vi "Lock VIs_V2.vi"() -> ()   [LabVIEW 2024]
panel:
  out "Errors":T1(array[cluster])
  in  "UnProtect All":bool
  in  "Protect All":bool
  out "Busy":bool
  in  "Reset":bool
  in  "Files":T2(array[cluster]) caption="Folder                                                                                Name                             Protected        Protect"
  in  "Unlock":bool
  in  "Lock":bool
  in  "Get Files":bool
  out "Locked Cnt":i32
  in  "Lock PW":string="KwestEng#8002"
  in  "Unlock PW":string
  in  "Folder":path
  # "Lock VIs Utility"
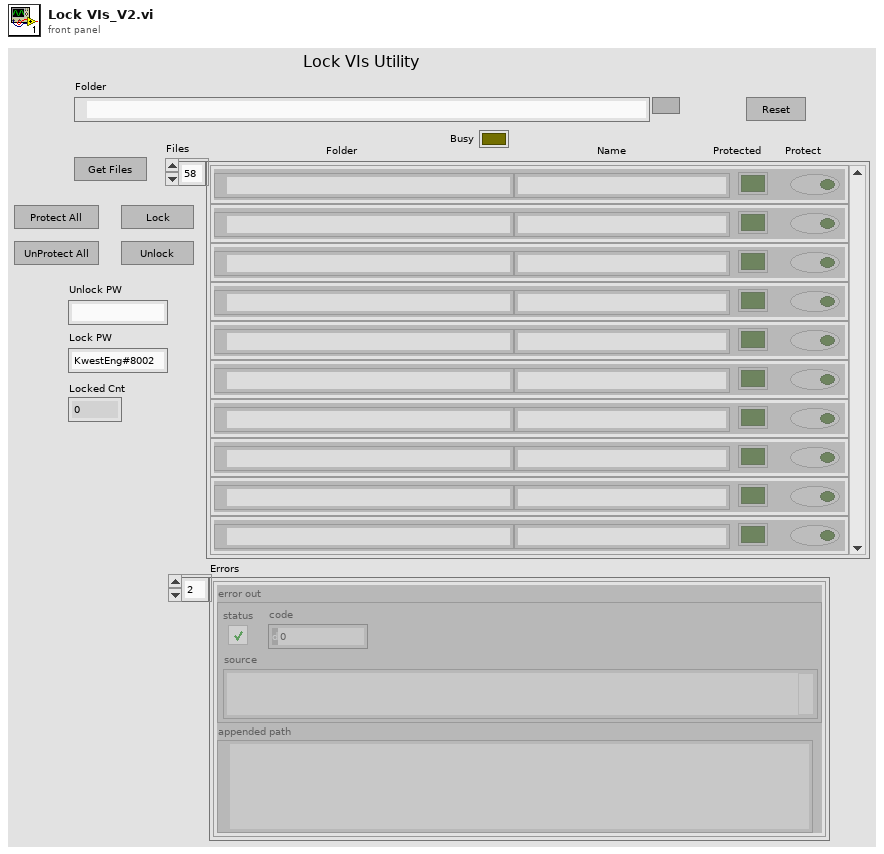
[diagram p1: front panel]
types:
  T1 = cluster{"error out":errorcluster, "appended path":path}[]
  T2 = cluster{"Name":string, "Folder":path, "Status":bool, "Protect":bool}[]
  T3 = enum32{"invalid app kind", "Development System", "Run Time System", "Student Edition", "Embedded LabVIEW", "Evaluation", "Custom"}
  T4 = cluster{"Name":string, "Folder":path, "Status":bool, "Protect":bool}
  T5 = enum32{"invalid lock state", "Not Locked", "Locked (No Password)", "Password-protected"}
  T6 = cluster{"Files":cluster{"Name":string, "Folder":path, "Status":bool, "Protect":bool}[], "UnlockPW":string, "LockPW":string}
  T7 = enum8{"Enabled", "Disabled", "Disabled and Grayed Out"}
  T8 = cluster{"error out":errorcluster, "appended path":path}
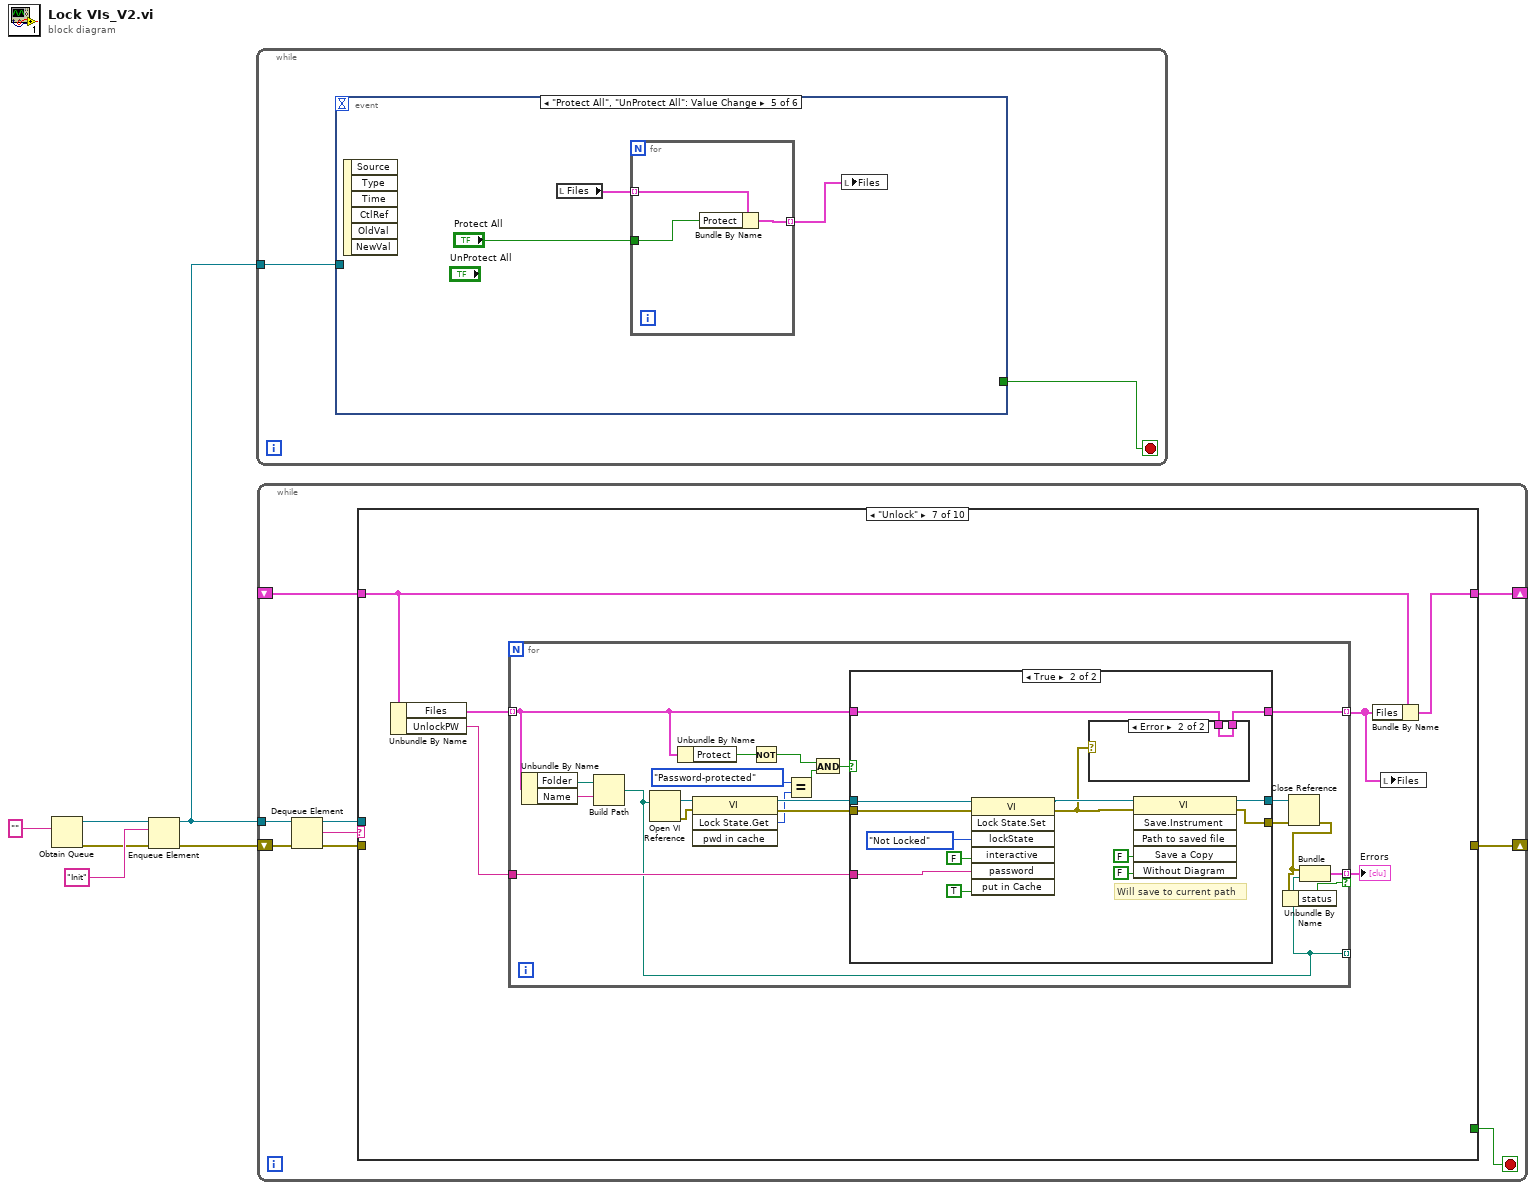
[diagram p0: block diagram]
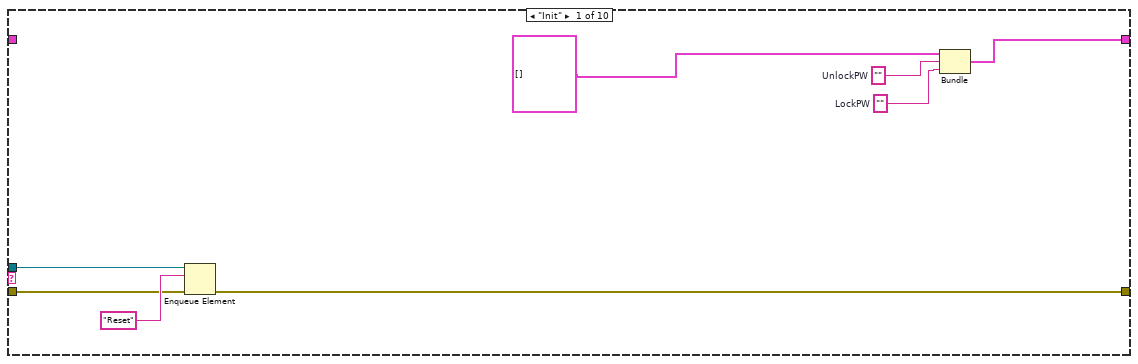
[diagram p2: hidden frame]
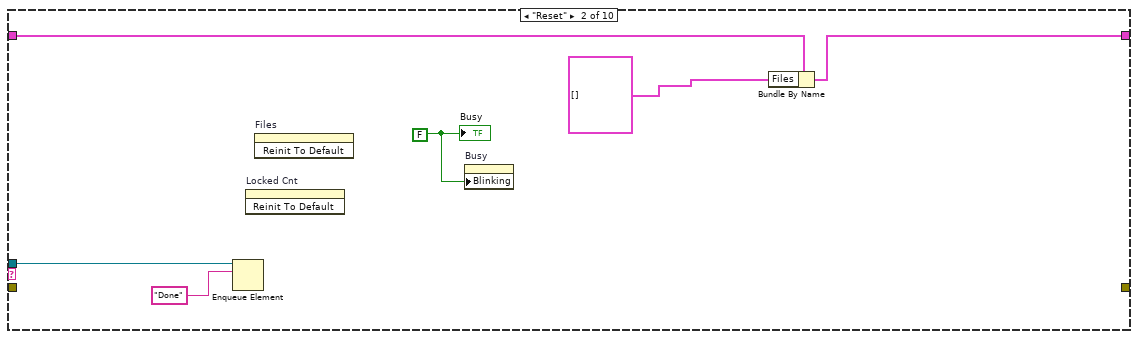
[diagram p3: hidden frame]
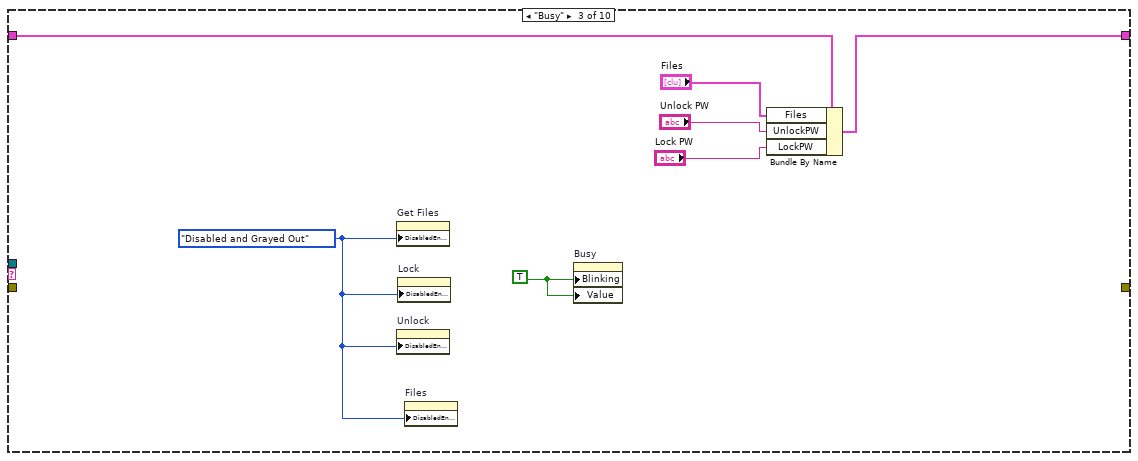
[diagram p4: hidden frame]
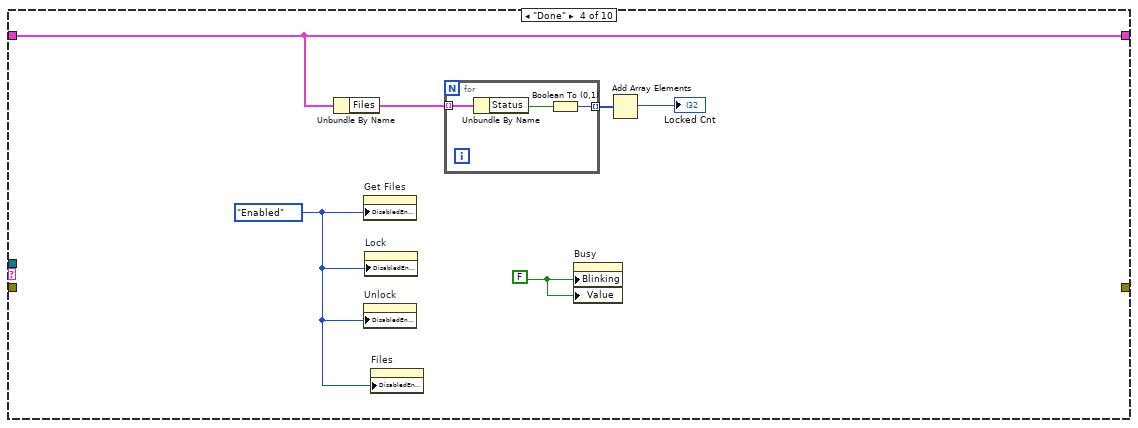
[diagram p5: hidden frame]
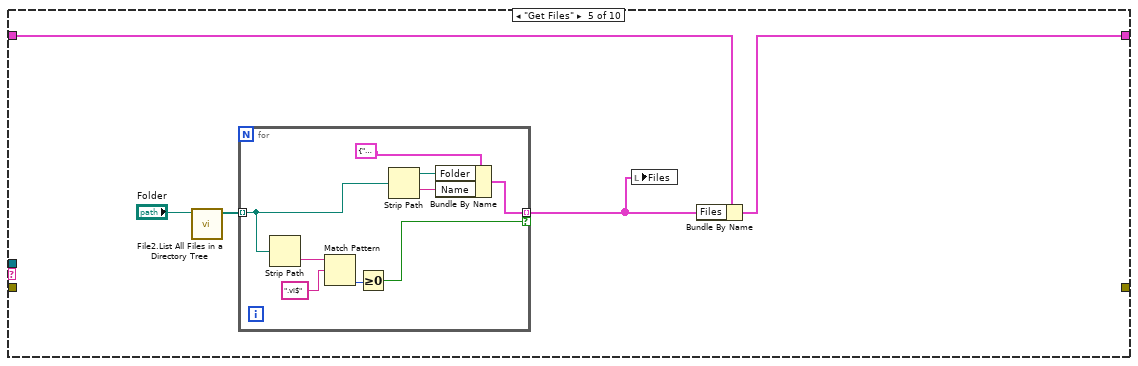
[diagram p6: hidden frame]
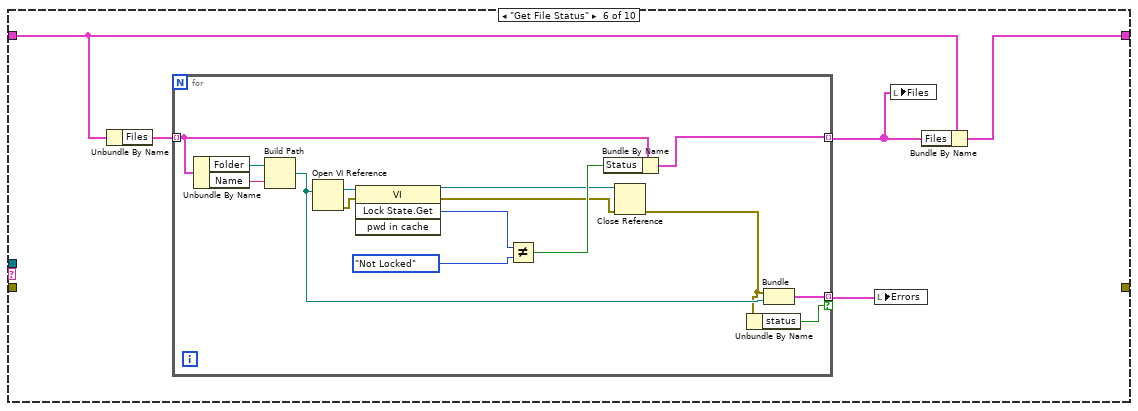
[diagram p7: hidden frame]
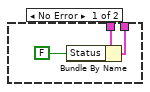
[diagram p9: hidden frame]
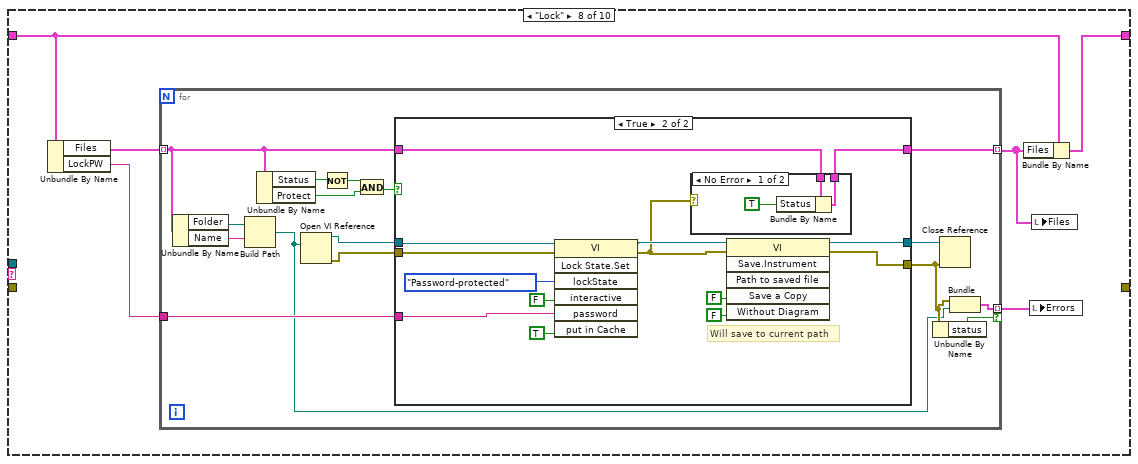
[diagram p10: hidden frame]
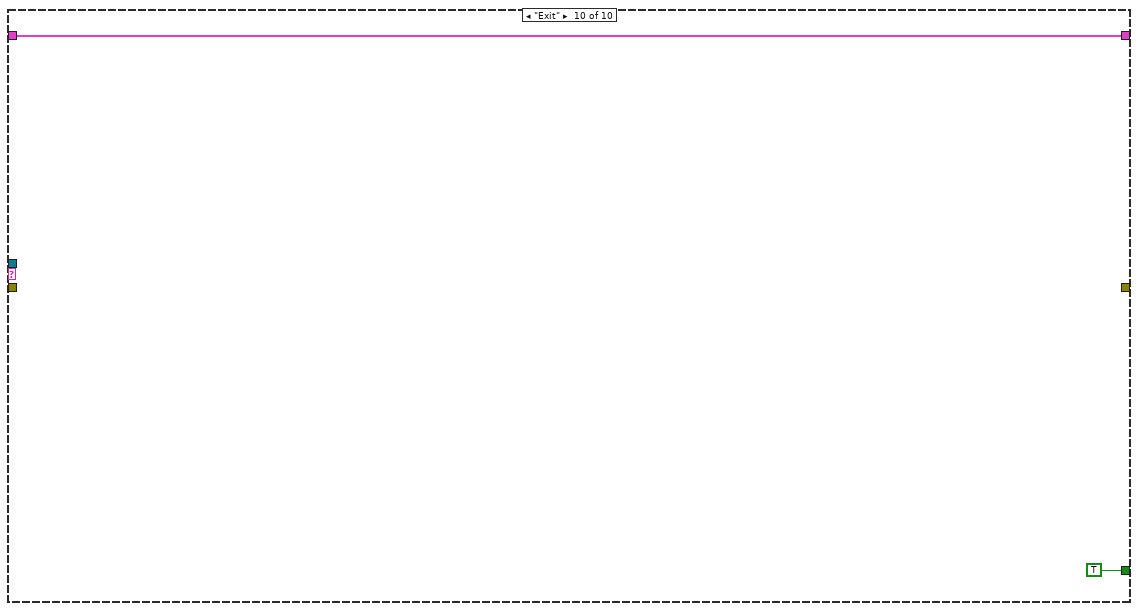
[diagram p14: hidden frame]
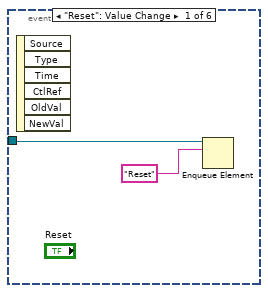
[diagram p15: hidden frame]
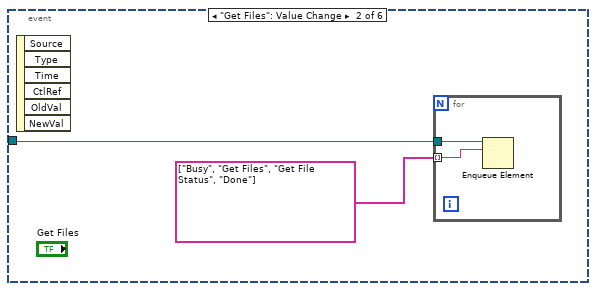
[diagram p16: hidden frame]
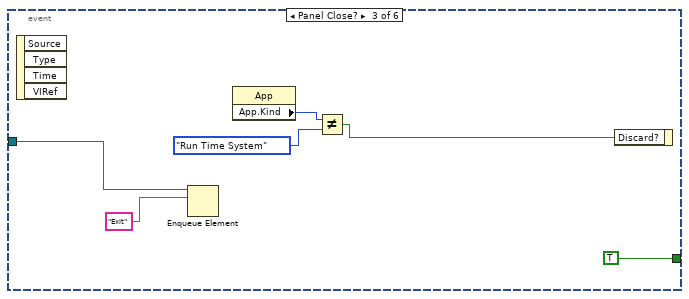
[diagram p17: hidden frame]
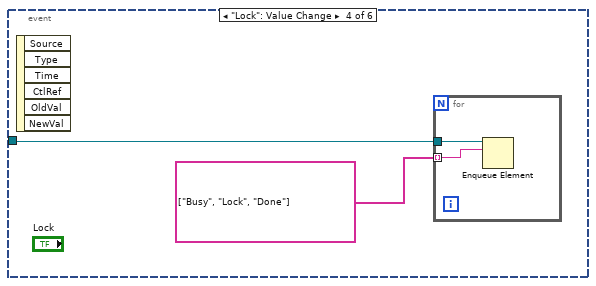
[diagram p18: hidden frame]
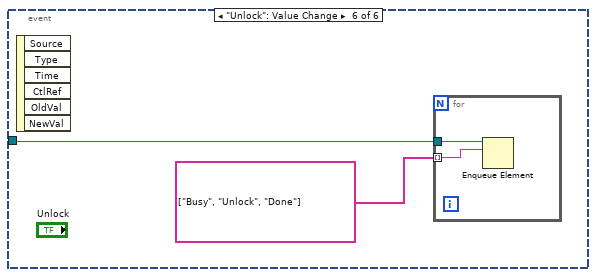
[diagram p19: hidden frame]
diagram:
  n1 = Obtain Queue(element data type="") -> (queue out=w4:refnum<queue>, error out=w1:errorcluster)  [unwired: 4 in, 1 out]
  n2 = Enqueue Element(queue=w4, element="Init", error in (no error)=w1) -> (queue out=w3:refnum<queue>, error out=w2:errorcluster)  [unwired: 1 in, 1 out]
  n3 = while {
    tunnel: w3 -> [w8]
    stop <- w7 stop-if-true
    n4 = event shown="[4] \"Protect All\", \"UnProtect All\": Value Change" {
      selector: _ -> [_ _ _ _ _ _]
      dyn-events: _ -> [_ _ _ _ _ _]
      timeout: _ -> [_ _ _ _ _ _]
      tunnel: w8 -> [w10 w12 w15 w22 _ w32]
      tunnel: [_ _ TRUE _ _ _] -> w7
      event "Reset": Value Change {
        n5 = event-data() -> ()  [unwired: 1 in, 6 out]
        n6 = Enqueue Element(queue=w10, element="Reset") -> ()  [unwired: 2 in, 3 out]
      }
      event "Get Files": Value Change {
        n7 = event-data() -> ()  [unwired: 1 in, 6 out]
        n8 = for {
          tunnel: w12 -> [w14]
          tunnel: string[] ["Busy", "Get Files", "Get File Status", "Done"] -> [w13] mode=indexing
          n9 = Enqueue Element(queue=w14, element=w13) -> ()  [unwired: 2 in, 3 out]
        }
      }
      event Panel Close? {
        n10 = event-data() -> ()  [unwired: 1 in, 4 out]
        n11 = Enqueue Element(queue=w15, element="Exit") -> ()  [unwired: 2 in, 3 out]
        n12 = property class="App"() -> ("App.Kind"=w19:T3)  [unwired: 2 in, 2 out]
        n13 = Not Equal?(x=w19, y=T3."Run Time System" ("Application:Kind")) -> (x != y?=w17:bool)
        n14 = event-data("Discard?"=w17) -> ()  [unwired: 1 in, 1 out]
      }
      event "Lock": Value Change {
        n15 = event-data() -> ()  [unwired: 1 in, 6 out]
        n16 = for {
          tunnel: w22 -> [w24]
          tunnel: string[] ["Busy", "Lock", "Done"] -> [w23] mode=indexing
          n17 = Enqueue Element(queue=w24, element=w23) -> ()  [unwired: 2 in, 3 out]
        }
      }
      event "Protect All", "UnProtect All": Value Change {
        n18 = event-data() -> ()  [unwired: 1 in, 6 out]
        n19 = local read "Files"() -> (w27:T2)
        n20 = for {
          tunnel: w27 -> [w30] mode=indexing
          tunnel: "Protect All" -> [w29]
          tunnel: [w28] -> w25 mode=indexing
          n21 = Bundle By Name(cluster=w30, "Protect"=w29) -> (w28:T4)
        }
        n22 = local write "Files"(w25) -> ()
      }
      event "Unlock": Value Change {
        n23 = event-data() -> ()  [unwired: 1 in, 6 out]
        n24 = for {
          tunnel: w32 -> [w34]
          tunnel: string[] ["Busy", "Unlock", "Done"] -> [w33] mode=indexing
          n25 = Enqueue Element(queue=w34, element=w33) -> ()  [unwired: 2 in, 3 out]
        }
      }
    }
  }
  n26 = while {
    tunnel: w3 -> [w42]
    shift-right: [w37] -> _
    shift-left: w2 -> [w39]
    shift-right: [w38] -> _
    shift-left: _ -> [w36]
    stop <- w35 stop-if-true
    n27 = Dequeue Element(queue=w42, error in (no error)=w39) -> (queue out=w43:refnum<queue>, element=w41:string, error out=w40:errorcluster)  [unwired: 1 in, 1 out]
    n28 = case shown="\"Unlock\"" w41 {
      tunnel: w43 -> [w47 w53 _ _ _ _ _ _ _ _]
      tunnel: w40 -> [w46 _ _ _ _ _ _ _ _ _]
      tunnel: [w51 w55 w60 w68 w75 w90 w110 w158 w199 w201] -> w38
      tunnel: [w45 _ _ _ _ _ _ _ _ _] -> w37
      tunnel: w36 -> [_ w56 w61 w68 w76 w91 w111 w159 w199 w201]
      tunnel: [_ _ _ _ _ _ _ _ _ TRUE] -> w35
      frame "Init" {
        w49 = ""  # LockPW
        w50 = ""  # UnlockPW
        n29 = Enqueue Element(queue=w47, element="Reset", error in (no error)=w46) -> (error out=w45:errorcluster)  [unwired: 1 in, 2 out]
        n30 = Bundle("Files"=T2 [], "UnlockPW"=w50, "LockPW"=w49) -> (w51:T6)  [unwired: 1 in]
      }
      frame "Reset" {
        w57 = FALSE
        n31 = Enqueue Element(queue=w53, element="Done") -> ()  [unwired: 2 in, 3 out]
        n32 = invoke on="Locked Cnt" class="DigNum (strict)" method="Reinit To Default"() -> ()  [unwired: 3 in, 3 out]
        n33 = invoke on="Files" class="Arr (strict)" method="Reinit To Default"() -> ()  [unwired: 3 in, 3 out]
        n34 = property on="Busy" class="Bool (strict)"("Blinking"=w57) -> ()  [unwired: 2 in, 2 out]
        n35 = Bundle By Name(cluster=w56, "Files"=T2 []) -> (w55:T6)
        "Busy" <- w57
      }
      frame "Busy" {
        w58 = T7."Disabled and Grayed Out" ("Disabled")
        w64 = TRUE
        n36 = property on="Get Files" class="Bool"("DisabledEnum"=w58) -> ()  [unwired: 2 in, 2 out]
        n37 = property on="Unlock" class="Bool"("DisabledEnum"=w58) -> ()  [unwired: 2 in, 2 out]
        n38 = property on="Lock" class="Bool"("DisabledEnum"=w58) -> ()  [unwired: 2 in, 2 out]
        n39 = property on="Files" class="Arr (strict)"("DisabledEnum"=w58) -> ()  [unwired: 2 in, 2 out]
        n40 = property on="Busy" class="Bool (strict)"("Blinking"=w64, "Value"=w64) -> ()  [unwired: 2 in, 2 out]
        n41 = Bundle By Name(cluster=w61, "Files"="Files", "UnlockPW"="Unlock PW", "LockPW"="Lock PW") -> (w60:T6)
      }
      frame "Done" {
        w69 = T7."Enabled" ("Disabled")
        w70 = FALSE
        n42 = Unbundle By Name(w68) -> ("Files"=w67:T2)
        n43 = property on="Get Files" class="Bool"("DisabledEnum"=w69) -> ()  [unwired: 2 in, 2 out]
        n44 = property on="Unlock" class="Bool"("DisabledEnum"=w69) -> ()  [unwired: 2 in, 2 out]
        n45 = property on="Lock" class="Bool"("DisabledEnum"=w69) -> ()  [unwired: 2 in, 2 out]
        n46 = property on="Files" class="Arr (strict)"("DisabledEnum"=w69) -> ()  [unwired: 2 in, 2 out]
        n47 = for {
          tunnel: w67 -> [w73] mode=indexing
          tunnel: [w71] -> w66 mode=indexing
          n48 = Unbundle By Name(w73) -> ("Status"=w72:bool)
          n49 = Boolean To (0,1)(Boolean=w72) -> (0, 1=w71:i16)
        }
        n50 = property on="Busy" class="Bool (strict)"("Blinking"=w70, "Value"=w70) -> ()  [unwired: 2 in, 2 out]
        n51 = Add Array Elements(numeric array=w66) -> (sum=→"Locked Cnt":i16)
      }
      frame "Get Files" {
        n52 = call "File2.List All Files in a Directory Tree.vi"("Folder"="Folder") -> ("Files"=w78:path[])  [unwired: 9 in, 1 out]
        n53 = for {
          tunnel: w78 -> [w80] mode=indexing
          tunnel: [w81] -> w74 mode=indexing if=w84
          n54 = Strip Path(path=w80) -> (name=w87:string)  [unwired: 1 out]
          n55 = Match Pattern(string=w87, regular expression=".vi$") -> (offset past match=w85:i32)  [unwired: 1 in, 3 out]
          n56 = Greater Or Equal To 0?(x=w85) -> (x >= 0?=w84:bool)
          n57 = Strip Path(path=w80) -> (stripped path=w83:path, name=w82:string)
          n58 = Bundle By Name(cluster=T4 {"Name"="", "Folder"=path "", "Status"=FALSE, "Protect"=FALSE} ("File Info"), "Folder"=w83, "Name"=w82) -> (w81:T4)
        }
        n59 = local write "Files"(w74) -> ()
        n60 = Bundle By Name(cluster=w76, "Files"=w74) -> (w75:T6)
      }
      frame "Get File Status" {
        n61 = Unbundle By Name(w91) -> ("Files"=w92:T2)
        n62 = for {
          tunnel: w92 -> [w106] mode=indexing
          tunnel: [w102] -> w89 mode=indexing
          tunnel: [w94] -> w88 mode=indexing if=w93
          n63 = Unbundle By Name(w106) -> ("Folder"=w100:path, "Name"=w99:string)
          n64 = Build Path(base path=w100, name or relative path=w99) -> (appended path=w97:path)
          n65 = Open VI Reference(vi path=w97) -> (vi reference=w107:refnum<vi>, error out=w98:errorcluster)  [unwired: 5 in]
          n66 = invoke class="VI" method="Lock State.Get"(reference=w107, error in=w98) -> (reference out=w101:refnum<vi>, error out=w96:errorcluster, "Get Lock State"=w104:T5)  [unwired: 2 in, 1 out]
          n67 = Not Equal?(x=w104, y=T5."Not Locked" ("Lock State:Get")) -> (x != y?=w103:bool)
          n68 = Bundle By Name(cluster=w106, "Status"=w103) -> (w102:T4)
          n69 = Close Reference(reference=w101, error in (no error)=w96) -> (error out=w95:errorcluster)
          n70 = Unbundle By Name(w95) -> ("status"=w93:bool)
          n71 = Bundle("error out"=w95, "appended path"=w97) -> (w94:T8)  [unwired: 1 in]
        }
        n72 = local write "Errors"(w88) -> ()
        n73 = local write "Files"(w89) -> ()
        n74 = Bundle By Name(cluster=w91, "Files"=w89) -> (w90:T6)
      }
      frame "Unlock" {
        n75 = Unbundle By Name(w111) -> ("Files"=w113:T2, "UnlockPW"=w112:string)
        n76 = for {
          tunnel: w113 -> [w125] mode=indexing
          tunnel: w112 -> [w128]
          tunnel: [w129] -> w109 mode=indexing
          tunnel: [w117] -> _ mode=indexing
          tunnel: [w116] -> w108 mode=indexing if=w114
          n77 = Unbundle By Name(w125) -> ("Folder"=w132:path, "Name"=w133:string)
          n78 = Build Path(base path=w132, name or relative path=w133) -> (appended path=w117:path)
          n79 = Open VI Reference(vi path=w117) -> (vi reference=w134:refnum<vi>, error out=w118:errorcluster)  [unwired: 5 in]
          n80 = Unbundle By Name(w125) -> ("Protect"=w122:bool)
          n81 = invoke class="VI" method="Lock State.Get"(reference=w134, error in=w118) -> (reference out=w131:refnum<vi>, error out=w127:errorcluster, "Get Lock State"=w124:T5)  [unwired: 2 in, 1 out]
          n82 = Not(x=w122) -> (.not. x?=w121:bool)
          n83 = Equal?(x=T5."Password-protected" ("Lock State"), y=w124) -> (x = y?=w120:bool)
          n84 = And(x=w121, y=w120) -> (x .and. y?=w119:bool)
          n85 = case shown="True" w119 {
            tunnel: w125 -> [w136 w145]
            tunnel: w131 -> [w137 w151]
            tunnel: [w137 w139] -> w130
            tunnel: [w136 w144] -> w129
            tunnel: w128 -> [_ w149]
            tunnel: w127 -> [w135 w146]
            tunnel: [w135 w140] -> w126
            frame False {
            }
            frame True {
              # "Will save to current path"
              n86 = invoke class="VI" method="Lock State.Set"(reference=w151, error in=w146, "lockState"=T5."Not Locked" ("Lock State"), "interactive"=FALSE ("Interactive"), "password"=w149, "put in Cache"=TRUE ("Put in Cache")) -> (reference out=w141:refnum<vi>, error out=w138:errorcluster)  [unwired: 1 in, 5 out]
              n87 = case shown="Error" w138 {
                tunnel: w145 -> [w154 w155]
                tunnel: [w153 w155] -> w144
                frame No Error {
                  n88 = Bundle By Name(cluster=w154, "Status"=FALSE) -> (w153:T4)
                }
                frame Error {
                }
              }
              n89 = invoke class="VI" method="Save.Instrument"(reference=w141, error in=w138, "Save a Copy"=FALSE, "Without Diagram"=FALSE) -> (reference out=w139:refnum<vi>, error out=w140:errorcluster)  [unwired: 2 in, 4 out]
            }
          }
          n90 = Close Reference(reference=w130, error in (no error)=w126) -> (error out=w115:errorcluster)
          n91 = Unbundle By Name(w115) -> ("status"=w114:bool)
          n92 = Bundle("error out"=w115, "appended path"=w117) -> (w116:T8)  [unwired: 1 in]
        }
        "Errors" <- w108
        n93 = Bundle By Name(cluster=w111, "Files"=w109) -> (w110:T6)
        n94 = local write "Files"(w109) -> ()
      }
      frame "Lock" {
        n95 = Unbundle By Name(w159) -> ("Files"=w161:T2, "LockPW"=w160:string)
        n96 = for {
          tunnel: w161 -> [w172] mode=indexing
          tunnel: w160 -> [w173]
          tunnel: [w174] -> w157 mode=indexing
          tunnel: [w163] -> w156 mode=indexing if=w162
          n97 = Unbundle By Name(w172) -> ("Folder"=w176:path, "Name"=w177:string)
          n98 = Build Path(base path=w176, name or relative path=w177) -> (appended path=w164:path)
          n99 = Unbundle By Name(w172) -> ("Status"=w169:bool, "Protect"=w166:bool)
          n100 = Open VI Reference(vi path=w164) -> (vi reference=w171:refnum<vi>, error out=w170:errorcluster)  [unwired: 5 in]
          n101 = Not(x=w169) -> (.not. x?=w168:bool)
          n102 = And(x=w168, y=w166) -> (x .and. y?=w167:bool)
          n103 = case shown="True" w167 {
            tunnel: w172 -> [w179 w183]
            tunnel: w171 -> [w180 w194]
            tunnel: [w180 w185] -> w175
            tunnel: [w179 w182] -> w174
            tunnel: w173 -> [_ w192]
            tunnel: w170 -> [w178 w189]
            tunnel: [w178 w184] -> w165
            frame False {
            }
            frame True {
              # "Will save to current path"
              n104 = invoke class="VI" method="Lock State.Set"(reference=w194, error in=w189, "lockState"=T5."Password-protected" ("Lock State"), "interactive"=FALSE ("Interactive"), "password"=w192, "put in Cache"=TRUE ("Put in Cache")) -> (reference out=w186:refnum<vi>, error out=w181:errorcluster)  [unwired: 1 in, 5 out]
              n105 = case shown="No Error" w181 {
                tunnel: w183 -> [w197 w198]
                tunnel: [w196 w198] -> w182
                frame No Error {
                  n106 = Bundle By Name(cluster=w197, "Status"=TRUE) -> (w196:T4)
                }
                frame Error {
                }
              }
              n107 = invoke class="VI" method="Save.Instrument"(reference=w186, error in=w181, "Save a Copy"=FALSE, "Without Diagram"=FALSE) -> (reference out=w185:refnum<vi>, error out=w184:errorcluster)  [unwired: 2 in, 4 out]
            }
          }
          n108 = Unbundle By Name(w165) -> ("status"=w162:bool)
          n109 = Close Reference(reference=w175, error in (no error)=w165) -> ()  [unwired: 1 out]
          n110 = Bundle("error out"=w165, "appended path"=w164) -> (w163:T8)  [unwired: 1 in]
        }
        n111 = Bundle By Name(cluster=w159, "Files"=w157) -> (w158:T6)
        n112 = local write "Errors"(w156) -> ()
        n113 = local write "Files"(w157) -> ()
      }
      frame "Error", Default {
      }
      frame "Exit" {
      }
    }
  }
